vi "Password Dialog.vi"(6 "Secret Type":T1=enum."Password", 7 "Address":string, 8 "Error In":errorcluster, 11 "Password In":string) -> (0 "Error Out":errorcluster, 3 "Password Out":string)   [LabVIEW 2017, in "Tests.lvlib"]
uses:
  Tests.lvlib
  Secret Types.ctl
  <vilib>/Utility/miscctls.llb/LVSelectionTypeDef.ctl
panel:
  out "Host":string="USERNAME FOR TEST SERVER"
  in  "Cancel":bool
  in  "OK":bool
  in  "Password":string
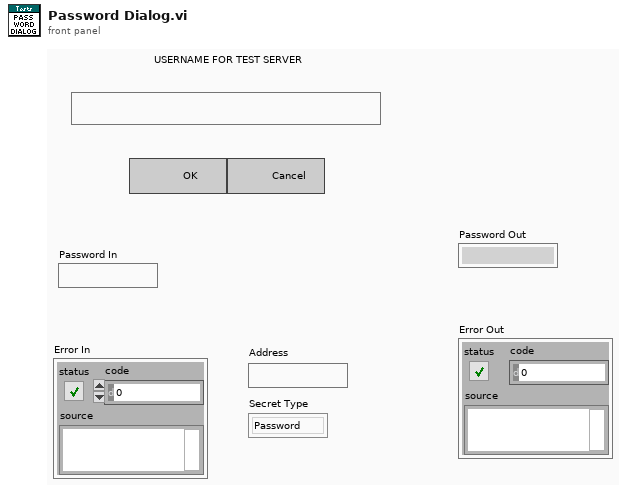
[diagram p1: front panel]
types:
  T1 = typedef "Tests.lvlib/Secret Types.ctl" = enum16{"Passphrase", "Password"}
  T2 = typedef "LVSelectionTypeDef.ctl" = cluster{"Selection Start":u32, "Selection End":u32}
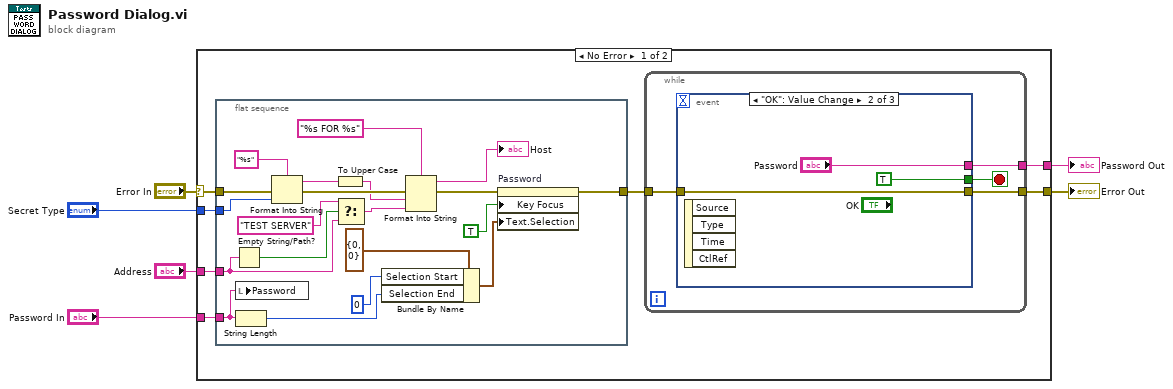
[diagram p0: block diagram]
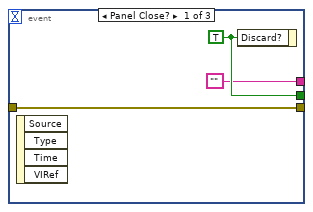
[diagram p2: hidden frame]
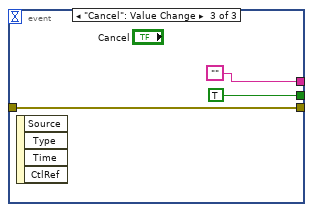
[diagram p3: hidden frame]
diagram:
  n1 = case shown="No Error" "Error In" {
    selector: "Error In" -> [w11 w47]
    tunnel: [w13 w47] -> w5
    tunnel: [w9 _] -> w4
    tunnel: "Password In" -> [w12 _]
    tunnel: "Address" -> [w8 _]
    tunnel: "Secret Type" -> [w7 _]
    frame No Error {
      n2 = flat-sequence {
        tunnel: w12 -> [w28]
        tunnel: w11 -> [w26]
        tunnel: [w33] -> w10
        tunnel: w8 -> [w21]
        tunnel: w7 -> [w17]
        frame #0 {
          n3 = Empty String/Path?(string/path=w21) -> (empty?=w22:bool)
          n4 = local write "Password"(w28) -> ()
          n5 = String Length(string=w28) -> (length=w27:i32)
          n6 = Format Into String(format string="%s", error in=w26, w17) -> (resulting string=w15:string, error out=w18:errorcluster)  [unwired: 1 in]
          n7 = To Upper Case(1:w15) -> (0:w14:string)
          n8 = Select(t="TEST SERVER", s=w22, f=w21) -> (s? t:f=w19:string)
          n9 = Bundle By Name(cluster=T2 {"Selection Start"=0, "Selection End"=0} ("Text.Selection"), "Selection Start"=u32 0, "Selection End"=w27) -> (w30:T2)
          n10 = Format Into String(format string="%s FOR %s", error in=w18, w14, w19) -> (resulting string=→"Host":string, error out=w25:errorcluster)  [unwired: 1 in]
          n11 = property on="Password" class="Str"(error in=w25, "Key Focus"=TRUE, "Text.Selection"=w30) -> (error out=w33:errorcluster)  [unwired: 1 in, 1 out]
        }
      }
      n12 = while {
        tunnel: w10 -> [w36]
        tunnel: [w35] -> w13
        tunnel: [w34] -> w9
        stop <- w37 stop-if-true
        n13 = event shown="[1] \"OK\": Value Change" {
          selector: _ -> [_ _ _]
          dyn-events: _ -> [_ _ _]
          timeout: _ -> [_ _ _]
          tunnel: [w40 TRUE TRUE] -> w37
          tunnel: w36 -> [w39 w43 w46]
          tunnel: [w39 w43 w46] -> w35
          tunnel: ["" "Password" ""] -> w34
          event Panel Close? {
            w40 = TRUE
            n14 = event-data() -> ()  [unwired: 1 in, 4 out]
            n15 = event-data("Discard?"=w40) -> ()  [unwired: 1 in, 1 out]
          }
          event "OK": Value Change {
            n16 = event-data() -> ()  [unwired: 1 in, 4 out]
          }
          event "Cancel": Value Change {
            n17 = event-data() -> ()  [unwired: 1 in, 4 out]
          }
        }
      }
    }
    frame Error {
    }
  }
  "Error Out" <- w5
  "Password Out" <- w4
